vi "ClimbNetwork.vi"   [LabVIEW 2020]
uses:
  ClimbGlobals.vi
  <vilib>/Rock Robotics/Network Tables/NT Write Number.vi
  <vilib>/Rock Robotics/Network Tables/NT Write Boolean.vi
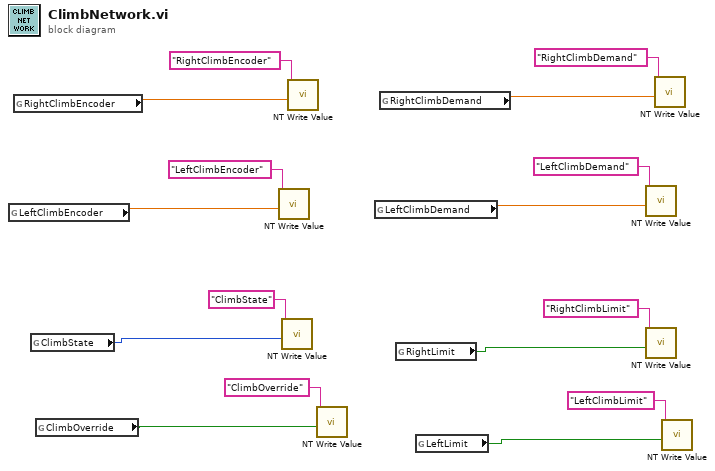
[diagram p0: block diagram]
diagram:
  n1 = global read "ClimbGlobals.vi" "LeftClimbEncoder"() -> (w11:dbl)
  n2 = global read "ClimbGlobals.vi" "RightClimbEncoder"() -> (w9:dbl)
  n3 = global read "ClimbGlobals.vi" "ClimbState"() -> (w15:i32)
  n4 = global read "ClimbGlobals.vi" "ClimbOverride"() -> (w13:bool)
  n5 = call-poly <vilib>:"NT Write Value.vi"("Numeric"=w11, "Name"="LeftClimbEncoder") -> ()  [unwired: 9 in, 1 out]
  n6 = call-poly <vilib>:"NT Write Value.vi"("Numeric"=w15, "Name"="ClimbState") -> ()  [unwired: 9 in, 1 out]
  n7 = call-poly <vilib>:"NT Write Value.vi"("Numeric"=w9, "Name"="RightClimbEncoder") -> ()  [unwired: 9 in, 1 out]
  n8 = call-poly <vilib>:"NT Write Value.vi"("Boolean"=w13, "Name"="ClimbOverride") -> ()  [unwired: 9 in, 1 out]
  n9 = global read "ClimbGlobals.vi" "LeftClimbDemand"() -> (w7:dbl)
  n10 = global read "ClimbGlobals.vi" "RightClimbDemand"() -> (w5:dbl)
  n11 = global read "ClimbGlobals.vi" "RightLimit"() -> (w3:bool)
  n12 = global read "ClimbGlobals.vi" "LeftLimit"() -> (w1:bool)
  n13 = call-poly <vilib>:"NT Write Value.vi"("Numeric"=w7, "Name"="LeftClimbDemand") -> ()  [unwired: 9 in, 1 out]
  n14 = call-poly <vilib>:"NT Write Value.vi"("Boolean"=w3, "Name"="RightClimbLimit") -> ()  [unwired: 9 in, 1 out]
  n15 = call-poly <vilib>:"NT Write Value.vi"("Numeric"=w5, "Name"="RightClimbDemand") -> ()  [unwired: 9 in, 1 out]
  n16 = call-poly <vilib>:"NT Write Value.vi"("Boolean"=w1, "Name"="LeftClimbLimit") -> ()  [unwired: 9 in, 1 out]
